vi "Send Message.vi"(8 "error in (no error)":errorcluster, 10 "Message":string, 11 "Connection Handler in":refnum<class "Connection Handler.lvclass">) -> (0 "error out":errorcluster, 3 "Connection Handler out":refnum<class "Connection Handler.lvclass">)   [LabVIEW 2017, in "Connection Handler.lvlib" / "Connection Handler.lvclass"]
uses:
  Connection Handler.lvclass
  Connection Handler.lvclass/Connection Handler.ctl
  <vilib>/MediaMongrels Ltd/WebSockets/Sockets/Socket/Socket.lvclass
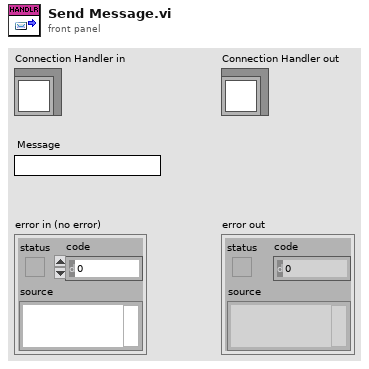
[diagram p1: front panel]
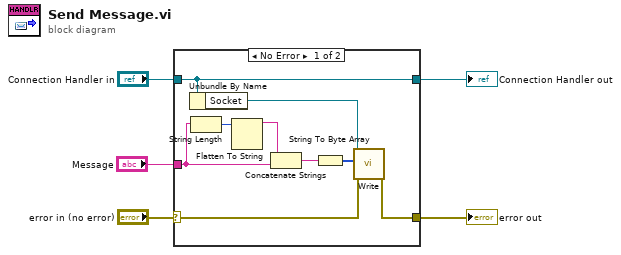
[diagram p0: block diagram]
diagram:
  n1 = case shown="No Error" "error in (no error)" {
    selector: "error in (no error)" -> [w12 w16]
    tunnel: [w11 w16] -> w4
    tunnel: [w14 w15] -> w2
    tunnel: "Connection Handler in" -> [w14 w15]
    tunnel: "Message" -> [w7 _]
    frame No Error {
      n2 = Unbundle By Name(w14) -> ("Socket"=w13:refnum<class "Socket.lvclass">)
      n3 = String Length(string=w7) -> (length=w10:i32)
      n4 = Flatten To String(anything=w10) -> (data string=w9:string)  [unwired: 1 in, 4 out]
      n5 = Concatenate Strings(w9, w7) -> (w8:string)
      n6 = String To Byte Array(string=w8) -> (unsigned byte array=w6:u8[])
      n7 = call-dynamic "Write.vi"("error in (no error)"=w12, "Bytes to write"=w6, "Socket in"=w13) -> ("error out"=w11:errorcluster)  [unwired: 6 in, 2 out]
    }
    frame Error {
    }
  }
  "error out" <- w4
  "Connection Handler out" <- w2
